vi "Gyro PID Fwd Dis WIND.vi"(6 "Target angle":sgl, 7 "Threshold to stop":i32=1200, 8 "Threshold to slow":i32=1000, 9 "Higher speed":i32=40, 10 "Max. speed":i32=80, 11 "EV3 in":T1) -> (3 "EV3 out":T1)   [LabVIEW 2015]
uses:
  <vilib>/NXT/Block Support/NXT_OutputPort.ctl
  <vilib>/NXT/LegoClasses/BrickReference/BrickReference.lvclass
  <vilib>/NXT/Subs/LVHSConnector.ctl
  <vilib>/NXT/NXTIO Xnodes/NXTIOXNode/NXTIO.xnode
  <vilib>/NXT/Dual Mode Library/Motors/Rotation.vi
  <vilib>/NXT/Dual Mode Library/Waits/Wait_Num.vi
  <vilib>/NXT/NXTIO Xnodes/NXTIONodeSubVIs/LEGOResetMotors.vi
  <vilib>/NXT/NXTIO Xnodes/NXTIONodeSubVIs/NXTMotorSteeringOn.vi
  <vilib>/NXT/NXTIO Xnodes/NXTIONodeSubVIs/NXTStopMotors.vi
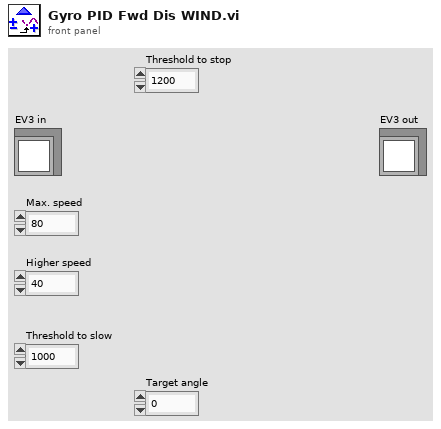
[diagram p1: front panel]
types:
  T1 = typedef "LVHSConnector.ctl" = refnum<class "BrickReference.lvclass">
  T2 = typedef "NXT_OutputPort.ctl" = u8
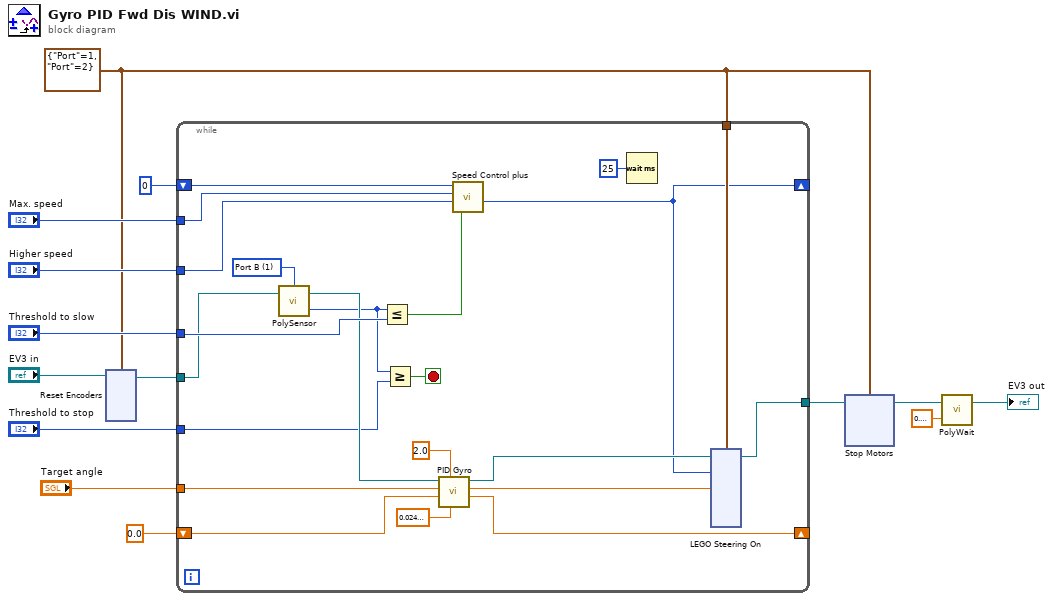
[diagram p0: block diagram]
diagram:
  w4 = cluster{"Port":T2, "Port":T2} {"Port"=1, "Port"=2} ("Motor")
  n1 = xnode "Reset Encoders"("Motors"=w4, "NXT/EV3"="EV3 in") -> ("NXT/EV3"=w10:T1)
  n2 = while {
    tunnel: w10 -> [w25]
    shift-right: [w36] -> _
    shift-left: sgl 0.0 -> [w19]
    tunnel: "Target angle" -> [w35]
    tunnel: [w32] -> w6
    tunnel: w4 -> [w34]
    shift-right: [w18] -> _
    shift-left: 0 -> [w29]
    tunnel: "Higher speed" -> [w26]
    tunnel: "Max. speed" -> [w28]
    tunnel: "Threshold to slow" -> [w27]
    tunnel: "Threshold to stop" -> [w17]
    stop <- w22 stop-if-true
    w33 = T2 1 items=["Port A", "Port B", "Port C", "Port D"] ("Port (Port A)")
    n3 = call-poly <vilib>:"PolySensor.vi"("NXT/EV3"=w25, "Port (Port A)"=w33) -> ("Angle of Rotation"=w21:i32, "NXT/EV3"=w24:T1)  [unwired: 1 in]
    n4 = Less Or Equal?(x=w21, y=w27) -> (x <= y?=w23:bool)
    n5 = Greater Or Equal?(x=w21, y=w17) -> (x >= y?=w22:bool)
    n6 = call "PID Gyro.vi"("K_i"=sgl 0.024, "K_p"=sgl 2.0, "Previous integral"=w19, "Target angle"=w35, "EV3 in"=w24) -> ("New integral"=w36:sgl, "Total error"=w30:sgl, "EV3 out"=w20:T1)  [unwired: 4 in]
    n7 = call "Speed Control plus.vi"("Speed Up or Down?"=w23, "Higher speed"=w26, "Max. speed"=w28, "Ini. speed"=w29) -> ("Speed out"=w18:i32)  [unwired: 7 in]
    n8 = Wait (ms)(milliseconds to wait=u32 25) -> ()  [unwired: 1 out]
    n9 = xnode "LEGO Steering On"("Steering 1"=w30, "Power 1"=w18, "Motors"=w34, "NXT/EV3"=w20) -> ("NXT/EV3"=w32:T1)
  }
  n10 = xnode "Stop Motors"("Motors"=w4, "NXT/EV3"=w6) -> ("NXT/EV3"=w5:T1)
  n11 = call-poly <vilib>:"PolyWait.vi"("Time (1 sec)"=sgl 0.2, "NXT/EV3"=w5) -> ("NXT/EV3"=→"EV3 out":T1)  [unwired: 2 in]
